vi "例4.5.vi"() -> ()   [LabVIEW 2018]
panel:
  in  "旋钮":dbl(knob) scale=0.0..10.0
  out "波形图表":dbl(graph)
  in  "控制开关":bool
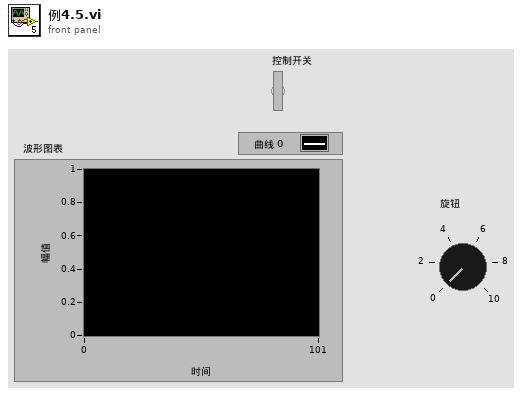
[diagram p1: front panel]
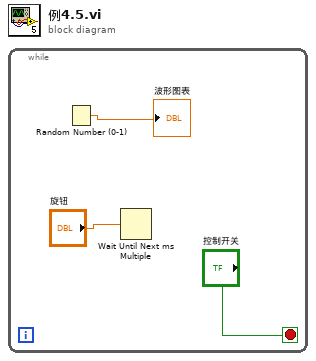
[diagram p0: block diagram]
diagram:
  n1 = while {
    stop <- "控制开关" stop-if-true
    n2 = Random Number (0-1)() -> (number: 0 to 1=→"波形图表":dbl)
    n3 = Wait Until Next ms Multiple(millisecond multiple="旋钮") -> ()  [unwired: 1 out]
  }
